vi "ShowErrorDialog.vi"(0 "reference in":refnum<class "MLA.lvclass">, 5 "error in (no error)":errorcluster) -> (14 "reference out":refnum<class "MLA.lvclass">, 19 "error out":errorcluster)   [LabVIEW 2017, in "MLA.lvclass"]
uses:
  MLA.lvclass
  S5Tools/ErrorLog/ErrorLog.lvclass
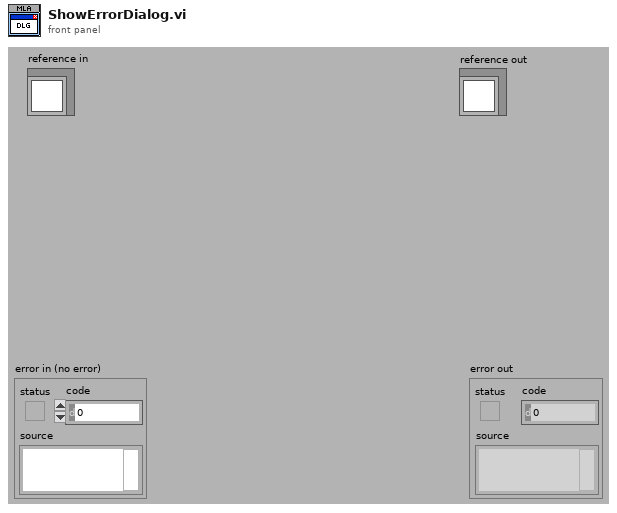
[diagram p1: front panel]
types:
  T1 = typedef "MLA.lvclass/ObjectAttributes.ctl" = cluster{"App Name":string, "App Version":string, "Revision History":string, "Log File Path":path, "Config INI File":path, "Config Path":path, "Log Archive Path":path, "Msg Q's":refnum<queue>[], "VI":refnum<vi>, "ErrLog":refnum<class "ErrorLog.lvclass">}
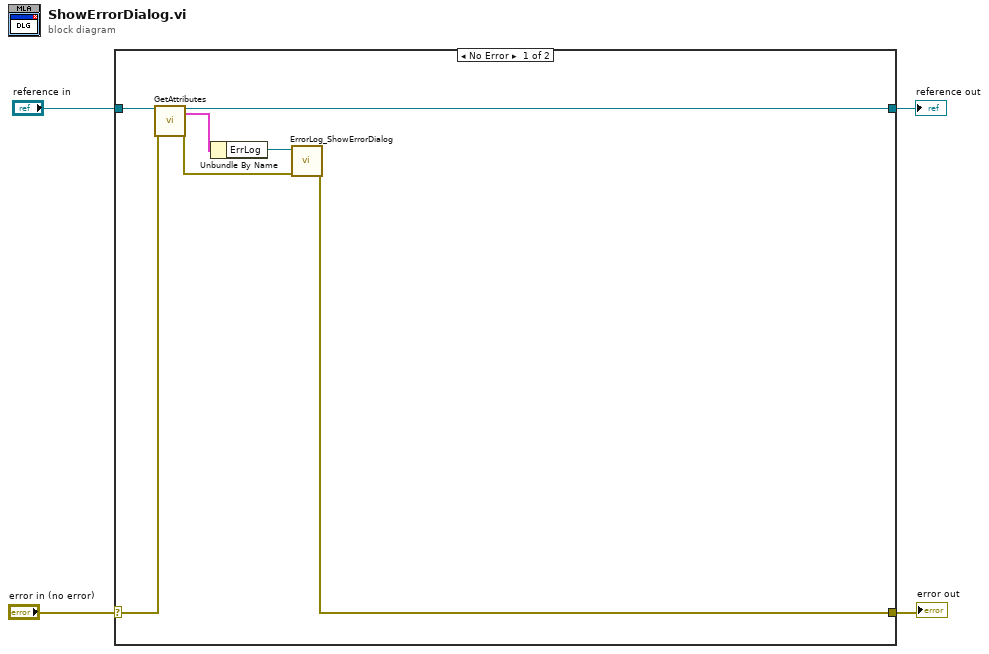
[diagram p0: block diagram]
diagram:
  n1 = case shown="No Error" "error in (no error)" {
    selector: "error in (no error)" -> [w11 w13]
    tunnel: [w5 w13] -> w3
    tunnel: [w8 w12] -> w1
    tunnel: "reference in" -> [w9 w12]
    frame No Error {
      n2 = call "GetAttributes.vi"("MLA"=w9, "error in (no error)"=w11) -> ("MLA"=w8:refnum<class "MLA.lvclass">, "Data"=w10:T1, "error out"=w6:errorcluster)  [unwired: 14 in, 1 out]
      n3 = Unbundle By Name(w10) -> ("ErrLog"=w7:refnum<class "ErrorLog.lvclass">)
      n4 = call-dynamic "ErrorLog_ShowErrorDialog.vi"("error in (no error)"=w6, "reference in"=w7) -> ("error out"=w5:errorcluster)  [unwired: 8 in, 1 out]
    }
    frame Error {
    }
  }
  "error out" <- w3
  "reference out" <- w1
